vi "GetPort.vi"(8 "error in (no error)":errorcluster, 10 "Port":u8, 11 "Simulated Device in":refnum<class "Simulated Device.lvclass">) -> (0 "error out":errorcluster, 1 "Response":string, 2 "Value":u8, 3 "Simulated Device out":refnum<class "Simulated Device.lvclass">)   [LabVIEW 2020, in "Simulated Device.lvclass"]
doc: "Get the status of a digital port on the target device."
uses:
  Simulated Device.lvclass
  Controls/Device Code.ctl
  Controls/Device Command Code.ctl
  <vilib>/Utility/error.llb/Error Cluster From Error Code.vi
  <vilib>/ErrorRing/Error Ring.xnode
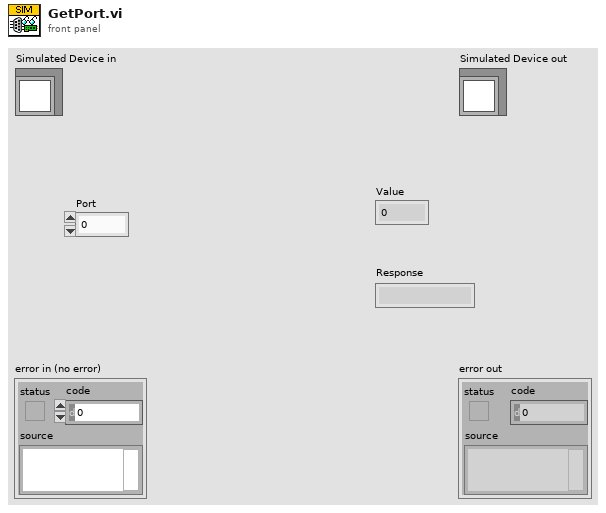
[diagram p1: front panel]
types:
  T1 = typedef "Device Command Code.ctl" = string
  T2 = typedef "Device Code.ctl" = string
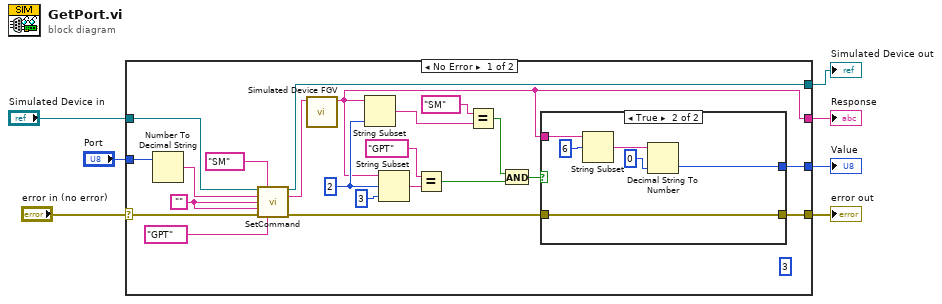
[diagram p0: block diagram]
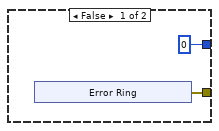
[diagram p2: hidden frame]
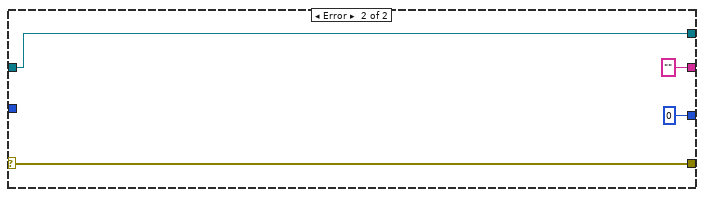
[diagram p3: hidden frame]
diagram:
  n1 = case shown="No Error" "error in (no error)" {
    selector: "error in (no error)" -> [w29 w45]
    tunnel: [w16 w45] -> w1
    tunnel: "Simulated Device in" -> [w27 w46]
    tunnel: [w23 w46] -> w4
    tunnel: "Port" -> [w25 _]
    tunnel: [w8 "" ("read buffer")] -> w2
    tunnel: [w12 u8 0] -> w3
    frame No Error {
      (unwired) 3 ("length (rest)")
      w21 = 2 ("length (rest)")
      w9 = "" ("Parameter 3")
      n2 = Number To Decimal String(number=w25) -> (decimal integer string=w24:string)  [unwired: 1 in]
      n3 = call-dynamic "SetCommand.vi"("Simulated Device in"=w27, "Device Code"=T2 "SM", "Parameter 1"=w24, "Parameter 2"=w9, "Parameter 3"=w9, "error in (no error)"=w29, "Command Code"=T1 "GPT") -> ("Simulated Device out"=w23:refnum<class "Simulated Device.lvclass">, "Command"=w10:string, "error out"=w11:errorcluster)  [unwired: 6 in]
      n4 = call "Simulated Device FGV.vi"("Request"=w10) -> ("Response"=w8:string)  [unwired: 10 in]
      n5 = String Subset(string=w8, length (rest)=w21) -> (substring=w14:string)  [unwired: 1 in]
      n6 = String Subset(string=w8, offset (0)=w21, length (rest)=3 ("length (rest)")) -> (substring=w22:string)
      n7 = Equal?(x=T1 "GPT" ("Command Code"), y=w22) -> (x = y?=w18:bool)
      n8 = Equal?(x=T2 "SM" ("Device Code"), y=w14) -> (x = y?=w15:bool)
      n9 = And(x=w15, y=w18) -> (x .and. y?=w17:bool)
      n10 = case shown="True" w17 {
        tunnel: w11 -> [_ w42]
        tunnel: [w31 w42] -> w16
        tunnel: w8 -> [_ w41]
        tunnel: [u8 0 w37] -> w12
        frame False {
          n11 = xnode "Error Ring"() -> ("error out"=w31:errorcluster)
        }
        frame True {
          n12 = String Subset(string=w41, offset (0)=6) -> (substring=w39:string)  [unwired: 1 in]
          n13 = Decimal String To Number(string=w39, default (0L)=u8 0 ("default (0 I32)")) -> (number=w37:u8)  [unwired: 1 in, 1 out]
        }
      }
    }
    frame Error {
    }
  }
  "error out" <- w1
  "Simulated Device out" <- w4
  "Response" <- w2
  "Value" <- w3
